vi "ColorizeGet.vi"(4 "error in (no error)":errorcluster, 6 "Container State":T4, 7 "Display State In":T1) -> (0 "error out":errorcluster, 2 "Value":bool, 3 "Display State Out":T1)   [LabVIEW 2013, in "VariantXControl__VP.xctl"]
uses:
  VariantXControl__VP.xctl
  <vilib>/_xctls/Container State.ctl
  VariantState.ctl
  Permissions.ctl
  TreeSettings.ctl
  <vilib>/_xctls/XControlSupport.lvlib
panel:
  # "Replace the Value Indicator below with an Indicator of desired type.\nDo not remove this Indicator or the others from the connector pane. \nDo not change the connector pane pattern.\nThe Value Indicator should always be the second terminal from top on the output side in the connector pane."
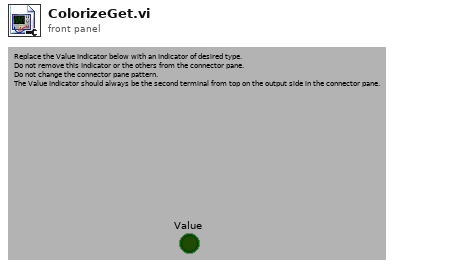
[diagram p1: front panel]
types:
  T1 = typedef "VariantXControl__VP.xctl/VariantState.ctl" = cluster{"State":string, "Messages":cluster{"Message":string, "Parameter":variant}[], "Current run":i32, "Start run":i32, "LastTag":string, "Tags":string[], "Length":i32, "Permissions":T2, "IsProbe?":bool, "Changed":bool, "TreeSettings":T3, "Tree Ref":refnum<vi>}
  T2 = typedef "VariantXControl__VP.xctl/Permissions.ctl" = cluster{"Reset":bool, "TraverseAttributes":bool, "Colorize":bool}
  T3 = typedef "VariantXControl__VP.xctl/TreeSettings.ctl" = cluster{"Traverse":bool, "Colorize":bool}
  T4 = typedef "XControlSupport.lvlib/Container State.ctl" = cluster{"Indicator?":bool, "Run Mode?":bool, " Refnum":refnum<vi>}
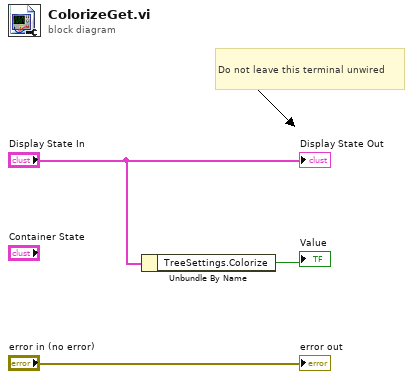
[diagram p0: block diagram]
diagram:
  # "Do not leave this terminal unwired"
  n1 = Unbundle By Name("Display State In") -> ("TreeSettings.Colorize"=→"Value":bool)
  "error out" <- "error in (no error)"
  "Display State Out" <- "Display State In"
